vi "Accumulated Correlation Function.vi"(9 "output selector":T1, 10 "data":T2, 11 "X":dbl[](array[numeric])) -> (0 "error out":errorcluster, 1 "inequality constraint function values":dbl[](array[numeric]), 2 "equality constraint function values":dbl[](array[numeric]), 3 "objective function value":dbl)   [LabVIEW 2012]
doc: "This template is the starting point for creating an objective function, equality constraint function and inequality constraint function to be passed to the Constrained Nonlinear Optimization.vi."
uses:
  <vilib>/gmath/NumericalOptimization/objective function data.ctl
  <vilib>/gmath/NumericalOptimization/cno_output select.ctl
  <vilib>/gmath/NI_Gmath.lvlib
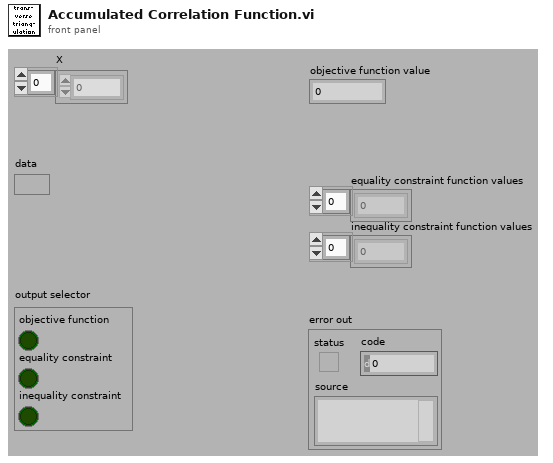
[diagram p1: front panel]
types:
  T1 = typedef "NI_Gmath.lvlib/cno_output select.ctl" = cluster{"objective function":bool, "equality constraint":bool, "inequality constraint":bool}
  T2 = typedef "NI_Gmath.lvlib/objective function data.ctl" = variant
  T3 = cluster{"Correlation Region\nSignal Waveforms":dbl[][], "Sampling Rate":i32, "Nr":i32, "Ntheta":i32, "Sensor Locations (cm)":dbl[][]}
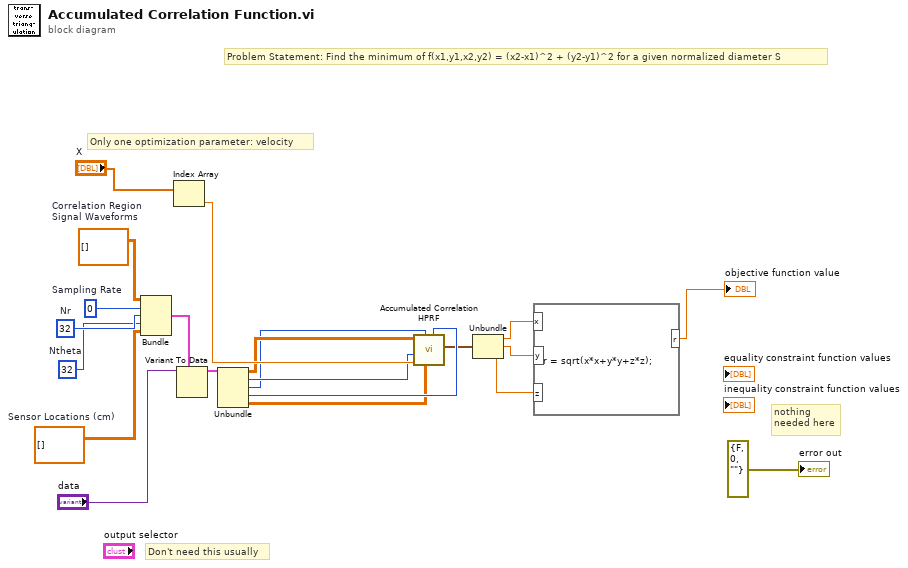
[diagram p0: block diagram]
diagram:
  w6 = dbl[][] []  # Sensor Locations (cm)
  w15 = 0  # Sampling Rate
  w11 = 32  # Ntheta
  w12 = 32  # Nr
  w19 = dbl[][] []  # Correlation Region Signal Waveforms
  # "nothing \nneeded here"
  # "Problem Statement: Find the minimum of f(x1,y1,x2,y2) = (x2-x1)^2 + (y2-y1)^2 for a given normalized diameter S"
  # "Don't need this usually"
  # "Only one optimization parameter: velocity"
  n1 = Bundle("Correlation Region\nSignal Waveforms"=w19, "Sampling Rate"=w15, "Nr"=w12, "Ntheta"=w11, "Sensor Locations (cm)"=w6) -> (w14:T3)  [unwired: 1 in]
  n2 = Index Array(array="X") -> (element=w16:dbl)  [unwired: 1 in]
  n3 = Variant To Data(type=w14, Variant="data") -> (data=w17:T3)  [unwired: 1 in, 1 out]
  n4 = Unbundle(w17) -> ("Correlation Region\nSignal Waveforms"=w13:dbl[][], "Sampling Rate"=w10:i32, "Nr"=w9:i32, "Ntheta"=w8:i32, "Sensor Locations (cm)"=w5:dbl[][])
  n5 = call "Accumulated Correlation HPRF.vi"("Ntheta"=w8, "Sensor Locations (cm)"=w5, "Nr"=w9, "Sound Velocity (cm/s)"=w16, "Sampling Rate"=w10, "Waveforms"=w13) -> ("Coordinates (m)"=w7:cluster{"x":dbl, "y":dbl, "z":dbl})  [unwired: 5 in]
  n6 = Unbundle(w7) -> ("x"=w4:dbl, "y"=w3:dbl, "z"=w2:dbl)
  n7 = formula code="r = sqrt(x*x+y*y+z*z);"("x"=w4, "y"=w3, "z"=w2) -> ("r"=→"objective function value":dbl)
  "error out" <- errorcluster {"status"=FALSE, "code"=0, "source"=""} ("error out")
